vi "PS_COND.vi"(0 "GUID":string) -> (2 "Cond (mS)":dbl, 3 "time date":string, 4 "File Path Out":path[](array[path]))   [LabVIEW 2019]
uses:
  5_Controls/PS_CMD_type-def.ctl
panel:
  in  "Cell Constant":dbl=0.485
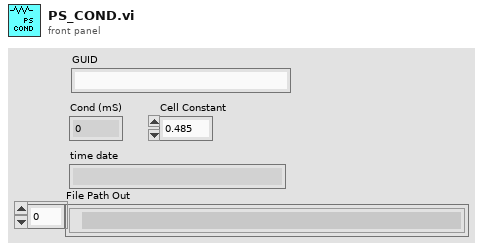
[diagram p1: front panel]
types:
  T1 = typedef "PS_CMD_type-def.ctl" = enum16{"Cond+Temp", "Cond_EIS", "Temp_EIS", "Vwind_MSP", "LongCond", "Cell1_EIS", "Cell2_EIS", "Cell3_EIS"}
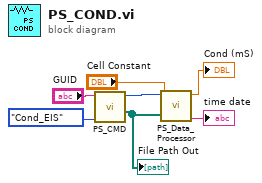
[diagram p0: block diagram]
diagram:
  n1 = call "PS_CMD.vi"(4:PS_CMD_type-def."Cond_EIS", "GUID"="GUID") -> ("File Path Out"=w5:path[], "Enum"=w6:T1)  [unwired: 4 in]
  "File Path Out" <- w5
  n2 = call "PS_Data_Processor.vi"("file path (dialog if empty)"=w5, "Cell Constant"="Cell Constant", 11:w6) -> ("time date"=→"time date":string, "Cond (mS)"=→"Cond (mS)":dbl)  [unwired: 2 in, 5 out]
